vi "SPU_Get_DeviceID.vi"(7 "错误输入（无错误）":errorcluster) -> (0 "error IO":errorcluster, 2 "id":string[](array[string]), 3 "引用输出":refnum<k24>)   [LabVIEW 2017]
doc: "Check Connction of spu deviece"
uses:
  D:/test/ILSTS/LV_IL_Sample/DLL/InstrumentDLL.dll
  DLL/InstrumentDLL.dll
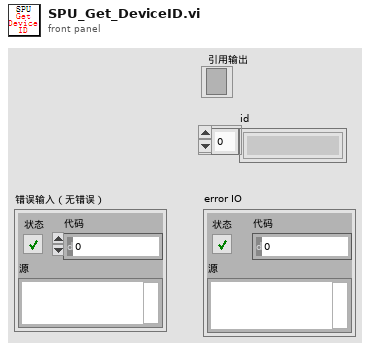
[diagram p1: front panel]
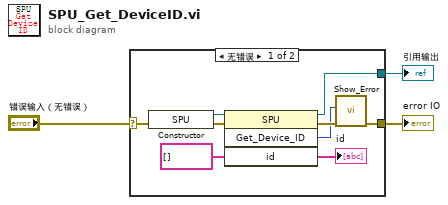
[diagram p0: block diagram]
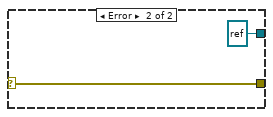
[diagram p2: hidden frame]
diagram:
  n1 = case shown="无错误" "错误输入（无错误）" {
    selector: "错误输入（无错误）" -> [w5 w14]
    tunnel: [w9 w14] -> w1
    tunnel: [w8 refnum<k24> refnum ("new reference")] -> w2
    frame No Error {
      n2 = constructor class="SPU"(error in=w5) -> (reference out=w6:refnum<k24>, error out=w4:errorcluster)  [unwired: 2 in, 1 out]
      n3 = invoke class="SPU" method="Get_Device_ID"(reference=w6, error in=w4, "id"=string[] []) -> (reference out=w8:refnum<k24>, error out=w11:errorcluster, "Get_Device_ID"=w10:i32, "id"=→"id":string[])  [unwired: 1 in]
      n4 = call "Show_Error.vi"("error in (no error)"=w11, "Error"=w10) -> ("error out"=w9:errorcluster)  [unwired: 9 in]
    }
    frame Error {
    }
  }
  "引用输出" <- w2
  "error IO" <- w1
